vi "take photo 52.vi"() -> ()   [LabVIEW 2019]
uses:
  <vilib>/myRIO/Instrument Drivers/Utilities/Utilities.lvlib
  <vilib>/myRIO/Common/Instrument Driver Framework/myRIO v1.0/DIO/typedefs/DIO Channels Enum.ctl
  <vilib>/myRIO/Common/Instrument Driver Framework/myRIO v1.0/DIO/typedefs/DIO Channels List.ctl
  <vilib>/myRIO/Common/Instrument Driver Framework/Utilities/typedefs/Generic FPGA Reference.ctl
  <vilib>/myRIO/Common/Instrument Driver Framework/Utilities/typedefs/myRIO v1.0 Reference.ctl
  <vilib>/myRIO/Common/Instrument Driver Framework/Utilities/typedefs/Hardware Version Enum.ctl
  <vilib>/myRIO/Common/Instrument Driver Framework/Utilities/typedefs/myRIO Generic Hardware Reference.ctl
  <vilib>/myRIO/Instrument Drivers/Onboard IO/DIO/typedefs/DIO Reference.ctl
  <vilib>/myRIO/Instrument Drivers/Onboard IO/DIO/DIO.lvlib
  <vilib>/myRIO/Instrument Drivers/Onboard IO/DIO/vis/Write.vi
  <vilib>/userDefined/High Color/nirio_resource_hc.ctl
  <vilib>/myRIO/Common/Instrument Driver Framework/myRIO v1.0/DIO/vis/myRIO v1.1 Open DIO.vi
  <vilib>/myRIO/Instrument Drivers/Onboard IO/DIO/vis/myRIO DIO Open.xnode
  <vilib>/myRIO/Common/Instrument Driver Framework/Utilities/vis/Is FPGA Ref Available.vi
  <vilib>/myRIO/Express VI/Onboard Devices/LED/LED Express VI.xnode
  <vilib>/myRIO/Instrument Drivers/Onboard IO/DIO/vis/Read.vi
  <vilib>/myRIO/Express VI/Onboard Devices/Button/Button Express VI.xnode
  sub/route_name.ctl
  subVI/move control/move and align/move_cluster.ctl
  sub/align position.ctl
panel:
  out "error out":errorcluster
  in  "Error In":errorcluster
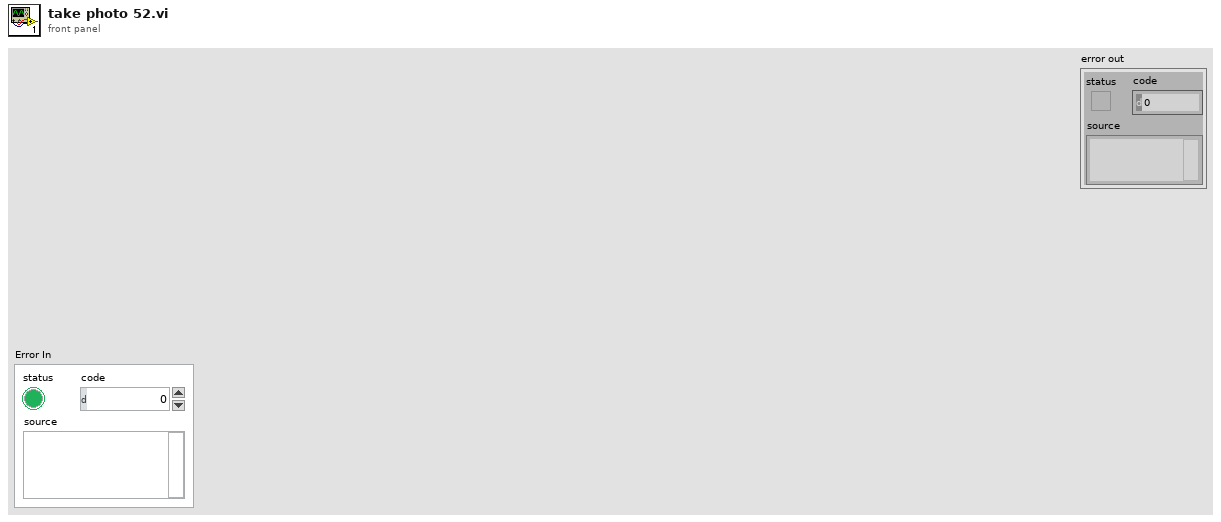
[diagram p1: front panel]
types:
  T1 = typedef "move_cluster.ctl" = cluster{"X":dbl, "Y":dbl, "degree":dbl, "speed":dbl}
  T2 = typedef "align position.ctl" = enum16{"S align", "vision align", "box align", "box to room align"}
  T3 = typedef "route_name.ctl" = enum16{"S-Vision", "Vision-R1", "Vision-R2", "Vision-R3", "Vision-R4", "Vision-R5", "R1-Vision", "R2-Vision", "R3-Vision", "R4-Vision", "R5-Vision", "Vision-box", "box-recycle", "recycle-box", "box-Vision", "Vision-S", "R2-R3"}
  T4 = typedef "DIO.lvlib/DIO Reference.ctl" = cluster{"myRIO Reference":T5, "DIO Channels List":T9}
  T5 = typedef "myRIO Generic Hardware Reference.ctl" = cluster{"myRIO Model":T6, "myRIO Hardware Reference":T7}
  T6 = typedef "Hardware Version Enum.ctl" = enum16{"Unknown", "myRIO-1900", "myRIO-1950", "roboRIO", "NI ELVIS RIO CM", "ELVIS III"}
  T7 = typedef "myRIO v1.0 Reference.ctl" = cluster{"Generic FPGA Reference":T8, "Allow multiple opens":bool}
  T8 = typedef "Generic FPGA Reference.ctl" = refnum<k20>
  T9 = typedef "DIO Channels List.ctl" = T10[]
  T10 = typedef "DIO Channels Enum.ctl" = enum16{"Not Connected", "C/DIO0", "C/DIO1", "C/DIO2", "C/DIO3", "C/DIO4", "C/DIO5", "C/DIO6", "C/DIO7", "A/DIO0", "A/DIO1", "A/DIO2", "A/DIO3", "A/DIO4", "A/DIO5", "A/DIO6", "A/DIO7", "A/DIO8", "A/DIO9", "A/DIO10", "A/DIO11", "A/DIO12", "A/DIO13", "A/DIO14", "A/DIO15", "A/DIO16", "A/DIO17", "A/DIO18", "A/DIO19", "B/DIO0", "B/DIO1", "B/DIO2", "B/DIO3", "B/DIO4", "B/DIO5", "B/DIO6", "B/DIO7", "B/DIO8", "B/DIO9", "B/DIO10", "B/DIO11", "B/DIO12", "B/DIO13", "B/DIO14", "B/DIO15", "B/DIO16", "B/DIO17", "B/DIO18", "B/DIO19", "LED0", "LED1", "LED2", "LED3", "Button0", "DIO/DIO0", "DIO/DIO1", "DIO/DIO2", "DIO/DIO3", "DIO/DIO4", "DIO/DIO5", "DIO/DIO6", "DIO/DIO7", "DIO/DIO8", "DIO/DIO9", "SPI/CS0", "SPI/CS1", "SPI/CS2", "SPI/CS3", "LED RADIO (Green)", "LED RADIO (Red)", "LED COMM (Green)", "LED COMM (Red)", "LED MODE (Green)", "LED MODE (Red)"}
  T11 = typedef "nirio_resource_hc.ctl" = tag
  T12 = typedef "position cluster.ctl" = cluster{"X":dbl, "Y":dbl, "Angle":dbl}
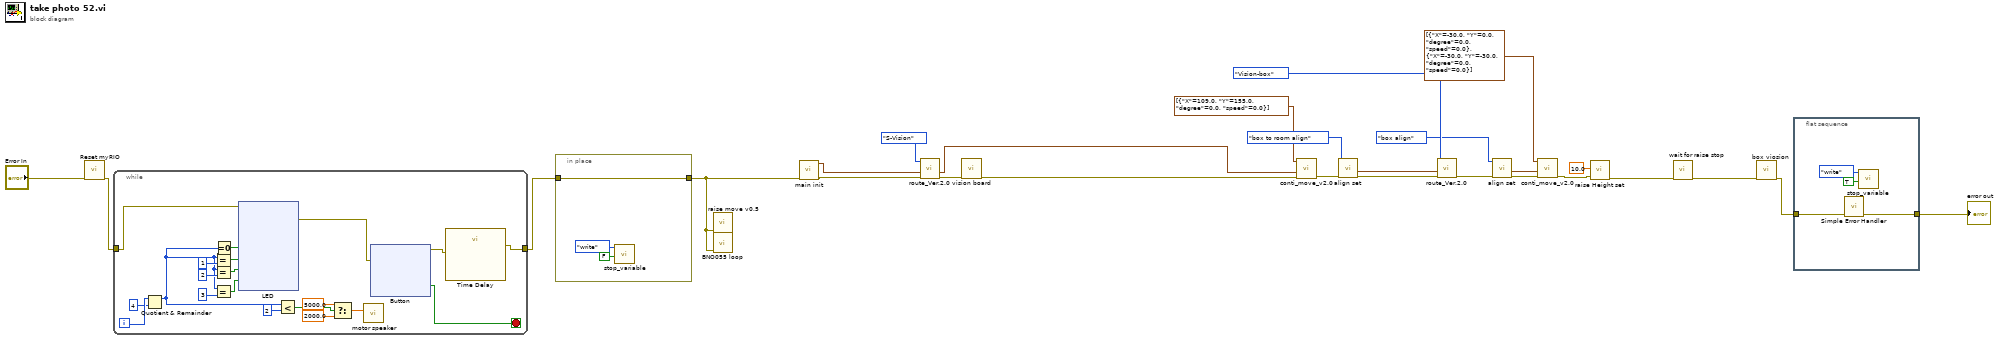
[diagram p0: block diagram]
diagram:
  n1 = call <vilib>:"Reset myRIO.vi"("error in (no error)"="Error In") -> ("error out"=w25:errorcluster)  [unwired: 10 in]
  n2 = while {
    tunnel: w25 -> [w38]
    tunnel: [w35] -> w24
    i -> [w47]
    stop <- w36 stop-if-true
    n3 = Quotient & Remainder(x=w47, y=4) -> (x-y*floor(x/y)=w33:i32)  [unwired: 1 out]
    n4 = Equal?(x=w33, y=1) -> (x = y?=w44:bool)
    n5 = Equal?(x=w33, y=2) -> (x = y?=w41:bool)
    n6 = Equal?(x=w33, y=3) -> (x = y?=w40:bool)
    n7 = Equal To 0?(x=w33) -> (x = 0?=w45:bool)
    n8 = xnode "LED"("LED0"=w45, "LED1"=w44, "LED2"=w41, "LED3"=w40, "error in (no error)"=w38) -> ("error out"=w37:errorcluster)
    n9 = Less?(x=w33, y=2) -> (x < y?=w30:bool)
    n10 = Select(t=5000.0, s=w30, f=2000.0) -> (s? t:f=w31:dbl)
    n11 = call "motor speaker.vi"("Vertical Pointer Slide"=w31) -> ()  [unwired: 11 in]
    n12 = xnode "Button"("error in (no error)"=w37) -> ("Value"=w36:bool, "error out"=w34:errorcluster)
    n13 = call "Time Delay"("error in (no error)"=w34) -> ("error out"=w35:errorcluster)  [unwired: 10 in]
  }
  n14 = in-place {
    in-place-border: [w123] -> w26
    in-place-border: w24 -> [w123]
    n15 = call "stop_variable.vi"("Write"=FALSE, "Enum"=enum16{"read", "write"}."write") -> ()  [unwired: 9 in, 1 out]
  }
  n16 = call "raise move v0.5.vi"("error in (no error)"=w26) -> ()  [unwired: 10 in, 1 out]
  n17 = call "BNO055 loop.vi"("error in (no error)"=w26) -> ()  [unwired: 11 in]
  n18 = call "main init.vi"("error in (no error)"=w26) -> ("error out"=w19:errorcluster, "position out"=w18:cluster{"x":dbl, "y":dbl, "degree":dbl})  [unwired: 9 in]
  n19 = call "route_Ver.2.0.vi"("error in (no error)"=w19, "Position"=w18, 11:route_name."S-Vision") -> ("error out"=w22:errorcluster, "Position out"=w21:T12)  [unwired: 7 in]
  n20 = call "vision board.vi"("error in (no error)"=w22) -> ("error out"=w20:errorcluster)  [unwired: 8 in, 2 out]
  n21 = call "conti_move_v2.0.vi"("error in (no error)"=w20, "Position"=w21, "route"=T1[] [{"X"=109.0, "Y"=155.0, "degree"=0.0, "speed"=0.0}]) -> ("error out"=w16:errorcluster)  [unwired: 7 in, 1 out]
  n22 = call "align set.vi"("error in (no error)"=w16, "align position"=align_position."box to room align") -> ("error out"=w14:errorcluster, "position out"=w13:cluster{"X":dbl, "y":dbl, "degree":dbl})  [unwired: 8 in]
  n23 = call "route_Ver.2.0.vi"("error in (no error)"=w14, "Position"=w13, 11:route_name."Vision-box") -> ("error out"=w10:errorcluster)  [unwired: 7 in, 1 out]
  n24 = call "align set.vi"("error in (no error)"=w10, "align position"=align_position."box align") -> ("error out"=w5:errorcluster, "position out"=w4:cluster{"X":dbl, "y":dbl, "degree":dbl})  [unwired: 8 in]
  n25 = call "conti_move_v2.0.vi"("error in (no error)"=w5, "Position"=w4, "route"=T1[] [{"X"=-30.0, "Y"=0.0, "degree"=0.0, "speed"=0.0}, {"X"=-30.0, "Y"=-30.0, "degree"=0.0, "speed"=0.0}]) -> ("error out"=w3:errorcluster)  [unwired: 7 in, 1 out]
  n26 = call "raise Height set.vi"("error in (no error)"=w3, "Height_cm"=10.0) -> ("error out"=w8:errorcluster)  [unwired: 9 in]
  n27 = call "wait for raise stop.vi"("Error In"=w8) -> ("Error Out"=w7:errorcluster)  [unwired: 10 in]
  n28 = call "box viosion.vi"("Error In"=w7) -> ("error out"=w2:errorcluster)  [unwired: 9 in, 1 out]
  n29 = flat-sequence {
    tunnel: w2 -> [w125]
    tunnel: [w124] -> w1
    frame #0 {
      n30 = call <vilib>:"Simple Error Handler.vi"("error in (no error)"=w125) -> ("error out"=w124:errorcluster)  [unwired: 4 in, 4 out]
      n31 = call "stop_variable.vi"("Write"=TRUE, "Enum"=enum16{"read", "write"}."write") -> ()  [unwired: 9 in, 1 out]
    }
  }
  "error out" <- w1
